vi "ExFileReadNGraphGbl.vi"() -> ()   [LabVIEW 2010]
panel:
  in  "Timeout":i16=1000
  out "FirstRunFlag":bool=TRUE
  in  "Quick Select":u32(knob) min=1 max=1000 scale=0.9..1.0
  in  "Set Position":bool
  out "Update Flag":bool=TRUE
  out "Waveform Graph":u16[](graph)
  in  "Spectrum Number":u32=1 min=1 step=1
  in  "Ending":bool
  in  "Beginning":bool
  out "Frame Number":i32=1
  in  "Backward":bool
  in  "Forward":bool
  in  "Full File Name":path=path "C:/Users/Public/Documents/SIToolKit/LabVIEW/Data Files/HID-LAMP.SPE"
  in  "Stop":bool
  in  "FileType":u32=67371008
  out "error out":errorcluster
  in  "error in (no error)":errorcluster
  # "NOTICE\n\nTHIS VI REQUIRES THAT THE TOOLKIT\nBE UNLOADED BY RUNNING THE\n VI EXCLOSEGLOBALCAM.VI\n BEFORE LEAVING LABVIEW."
  # "ExReadFileNGraphGbl.vi\nThis example will read in a file of the\nselected data type and display all frames.\nWhen finished viewing data, make sure to\nuse the STOP button to close the display."
  # "File Types:\nSPE = 67371008\nTIF   = 67174400\nPMI  = 67436544"
  # "Browse match pattern is set to *.tif.  Modify this if different file type is needed."
  # "This will properly \ndeallocate memory."
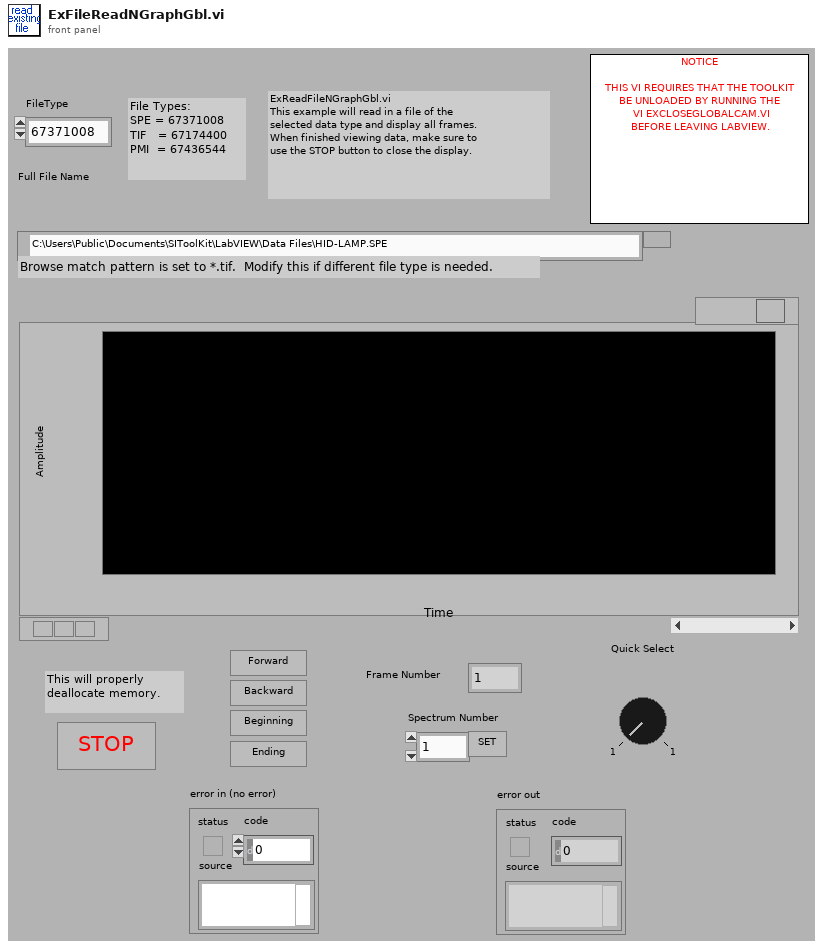
[diagram p1: front panel]
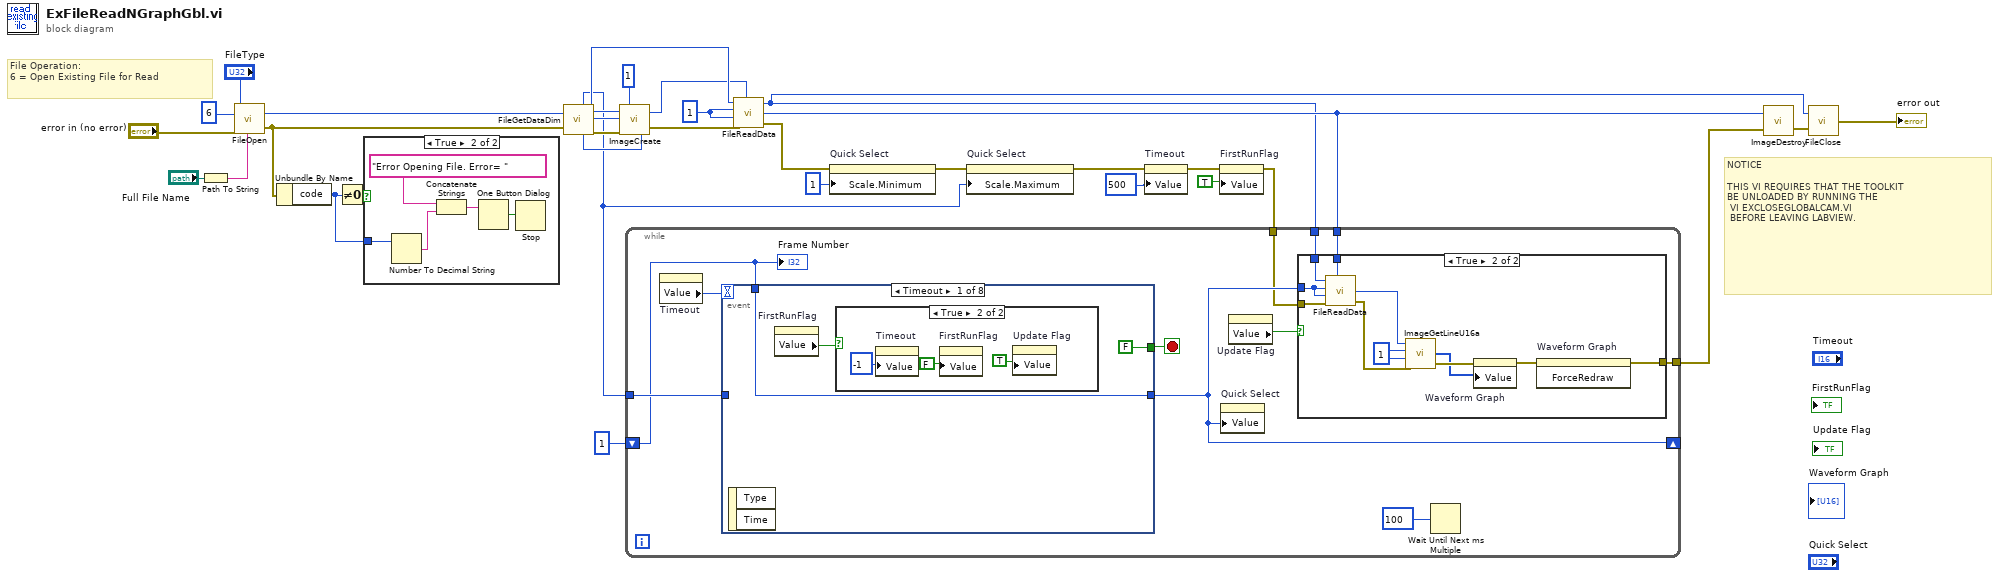
[diagram p0: block diagram]
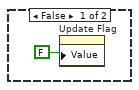
[diagram p3: hidden frame]
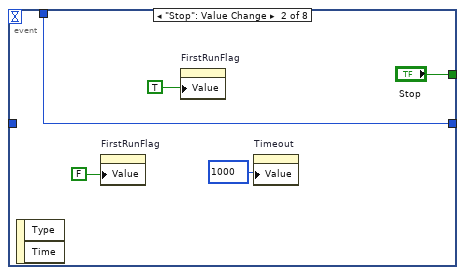
[diagram p4: hidden frame]
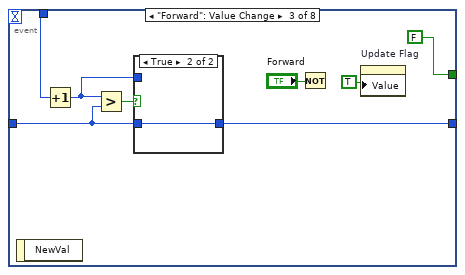
[diagram p5: hidden frame]
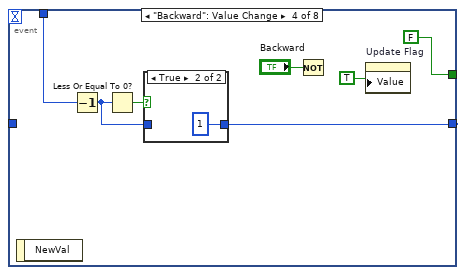
[diagram p7: hidden frame]
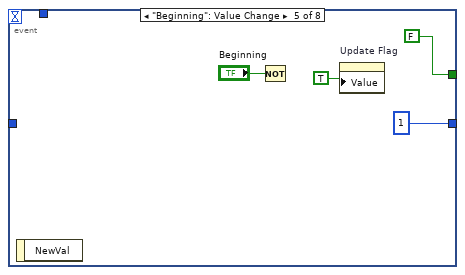
[diagram p9: hidden frame]
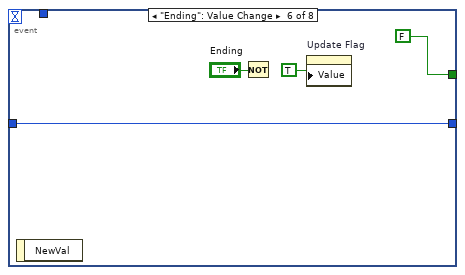
[diagram p10: hidden frame]
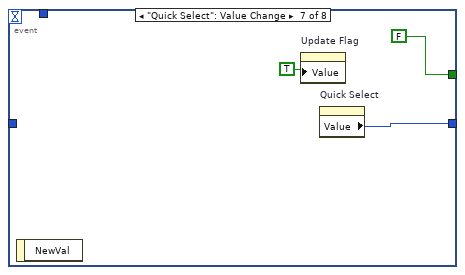
[diagram p11: hidden frame]
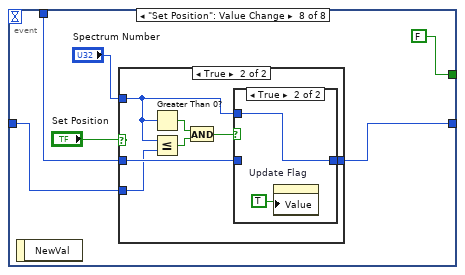
[diagram p12: hidden frame]
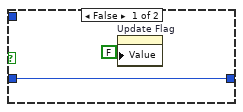
[diagram p13: hidden frame]
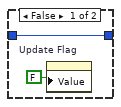
[diagram p14: hidden frame]
diagram:
  w20 = 1
  # "NOTICE\n\nTHIS VI REQUIRES THAT THE TOOLKIT\nBE UNLOADED BY RUNNING THE\n VI EXCLOSEGLOBALCAM.VI\n BEFORE LEAVING LABVIEW."
  # "File Operation:\n6 = Open Existing File for Read"
  n1 = Path To String(path="Full File Name") -> (string=w23:string)
  n2 = call <userlib>:"FileOpen.vi"("error in"="error in (no error)", "File Operations"=u32 6 ("File Operation"), "FileName"=w23, "File Type"="FileType") -> ("error out"=w12:errorcluster, "File Handle"=w17:u32)
  n3 = Unbundle By Name(w12) -> ("code"=w10:i32)
  n4 = Not Equal To 0?(x=w10) -> (x != 0?=w11:bool)
  n5 = case shown="True" w11 {
    tunnel: w10 -> [_ w34]
    frame False {
    }
    frame True {
      n6 = Number To Decimal String(number=w34) -> (decimal integer string=w35:string)  [unwired: 1 in]
      n7 = Concatenate Strings("Error Opening File. Error= ", w35) -> (w37:string)
      n8 = One Button Dialog(message=w37) -> (true=w36:bool)  [unwired: 1 in]
      n9 = Stop(stop? (T)=w36) -> ()
    }
  }
  n10 = call <userlib>:"FileGetDataDim.vi"("File Handle"=w17, "error in"=w12) -> ("Number of Frames"=w6:u32, "Data Type"=w27:u32, "File Handle"=w19:u32, "X dim"=w29:u32, "Y dim"=w28:u32, "error out"=w30:errorcluster)
  n11 = call <userlib>:"ImageCreate.vi"("X dimension"=w29, "Y dimension"=w28, "Data Type"=w27, "error in"=w30, "Number Of Frames"=1) -> ("Image Handle"=w18:u32, "error out"=w13:errorcluster)
  n12 = call <userlib>:"FileReadData.vi"("File Handle"=w19, "Start Frame"=w20, "End Frame"=w20, "error in"=w13, "Image Handle"=w18) -> ("File Handle"=w15:u32, "Image Handle"=w16:u32, "error out"=w8:errorcluster)
  n13 = property on="Quick Select" class="Knob (strict)"(error in=w8, "Scale.Minimum"=1) -> (error out=w9:errorcluster)  [unwired: 1 in, 1 out]
  n14 = property on="Quick Select" class="Knob (strict)"(error in=w9, "Scale.Maximum"=w6) -> (error out=w5:errorcluster)  [unwired: 1 in, 1 out]
  n15 = property on="Timeout" class="DigNum (strict)"(error in=w5, "Value"=500) -> (error out=w3:errorcluster)  [unwired: 1 in, 1 out]
  n16 = property on="FirstRunFlag" class="Bool (strict)"(error in=w3, "Value"=TRUE) -> (error out=w2:errorcluster)  [unwired: 1 in, 1 out]
  n17 = while {
    shift-right: [w42] -> _
    shift-left: 1 -> [w44]
    tunnel: w2 -> [w39]
    tunnel: w15 -> [w48]
    tunnel: w16 -> [w47]
    tunnel: [w49] -> w14
    tunnel: w6 -> [w45]
    stop <- w43 stop-if-true
    n18 = property on="Timeout" class="DigNum (strict)"() -> ("Value"=w41:i16)  [unwired: 2 in, 2 out]
    n19 = event shown="[0] Timeout" {
      selector: _ -> [_ _ _ _ _ _ _ _]
      dyn-events: _ -> [_ _ _ _ _ _ _ _]
      timeout: w41 -> [_ _ _ _ _ _ _ _]
      tunnel: w45 -> [_ _ w67 _ _ w87 _ w96]
      tunnel: w44 -> [w52 w60 w66 w76 _ _ _ w95]
      tunnel: [w52 w60 w65 w75 1 w87 w90 w93] -> w42
      tunnel: [FALSE "Stop" FALSE FALSE FALSE FALSE FALSE FALSE] -> w43
      event Timeout {
        n20 = event-data() -> ()  [unwired: 1 in, 2 out]
        n21 = property on="FirstRunFlag" class="Bool (strict)"() -> ("Value"=w50:bool)  [unwired: 2 in, 2 out]
        n22 = case shown="True" w50 {
          frame False {
            n23 = property on="Update Flag" class="Bool (strict)"("Value"=FALSE) -> ()  [unwired: 2 in, 2 out]
          }
          frame True {
            n24 = property on="Timeout" class="DigNum (strict)"("Value"=-1) -> ()  [unwired: 2 in, 2 out]
            n25 = property on="FirstRunFlag" class="Bool (strict)"("Value"=FALSE) -> ()  [unwired: 2 in, 2 out]
            n26 = property on="Update Flag" class="Bool (strict)"("Value"=TRUE) -> ()  [unwired: 2 in, 2 out]
          }
        }
      }
      event "Stop": Value Change {
        n27 = event-data() -> ()  [unwired: 1 in, 2 out]
        n28 = property on="FirstRunFlag" class="Bool (strict)"("Value"=FALSE) -> ()  [unwired: 2 in, 2 out]
        n29 = property on="FirstRunFlag" class="Bool (strict)"("Value"=TRUE) -> ()  [unwired: 2 in, 2 out]
        n30 = property on="Timeout" class="DigNum (strict)"("Value"=1000) -> ()  [unwired: 2 in, 2 out]
      }
      event "Forward": Value Change {
        n31 = event-data() -> ()  [unwired: 1 in, 1 out]
        n32 = Increment(x=w66) -> (x+1=w68:u32)
        n33 = Greater?(x=w68, y=w67) -> (0:w69:bool)
        n34 = case shown="True" w69 {
          tunnel: w67 -> [_ w71]
          tunnel: [w70 w71] -> w65
          tunnel: w68 -> [w70 _]
          frame False {
          }
          frame True {
          }
        }
        n35 = Not(x="Forward") -> ()  [unwired: 1 out]
        n36 = property on="Update Flag" class="Bool (strict)"("Value"=TRUE) -> ()  [unwired: 2 in, 2 out]
      }
      event "Backward": Value Change {
        n37 = event-data() -> ()  [unwired: 1 in, 1 out]
        n38 = Decrement(x=w76) -> (x-1=w77:u32)
        n39 = Less Or Equal To 0?(x=w77) -> (x <= 0?=w78:bool)
        n40 = case shown="True" w78 {
          tunnel: [w79 1] -> w75
          tunnel: w77 -> [w79 _]
          frame False {
          }
          frame True {
          }
        }
        n41 = Not(x="Backward") -> ()  [unwired: 1 out]
        n42 = property on="Update Flag" class="Bool (strict)"("Value"=TRUE) -> ()  [unwired: 2 in, 2 out]
      }
      event "Beginning": Value Change {
        n43 = event-data() -> ()  [unwired: 1 in, 1 out]
        n44 = Not(x="Beginning") -> ()  [unwired: 1 out]
        n45 = property on="Update Flag" class="Bool (strict)"("Value"=TRUE) -> ()  [unwired: 2 in, 2 out]
      }
      event "Ending": Value Change {
        n46 = event-data() -> ()  [unwired: 1 in, 1 out]
        n47 = Not(x="Ending") -> ()  [unwired: 1 out]
        n48 = property on="Update Flag" class="Bool (strict)"("Value"=TRUE) -> ()  [unwired: 2 in, 2 out]
      }
      event "Quick Select": Value Change {
        n49 = event-data() -> ()  [unwired: 1 in, 1 out]
        n50 = property on="Update Flag" class="Bool (strict)"("Value"=TRUE) -> ()  [unwired: 2 in, 2 out]
        n51 = property on="Quick Select" class="Knob (strict)"() -> ("Value"=w90:u32)  [unwired: 2 in, 2 out]
      }
      event "Set Position": Value Change {
        n52 = event-data() -> ()  [unwired: 1 in, 1 out]
        n53 = case shown="True" "Set Position" {
          tunnel: w95 -> [w99 w101]
          tunnel: [w99 w102] -> w93
          tunnel: "Spectrum Number" -> [_ w103]
          tunnel: w96 -> [_ w100]
          frame False {
            n54 = property on="Update Flag" class="Bool (strict)"("Value"=FALSE) -> ()  [unwired: 2 in, 2 out]
          }
          frame True {
            n55 = Greater Than 0?(x=w103) -> (x > 0?=w105:bool)
            n56 = Less Or Equal?(x=w103, y=w100) -> (x <= y?=w104:bool)
            n57 = And(x=w105, y=w104) -> (x .and. y?=w106:bool)
            n58 = case shown="True" w106 {
              tunnel: w103 -> [_ w110]
              tunnel: [w108 w110] -> w102
              tunnel: w101 -> [w108 _]
              frame False {
                n59 = property on="Update Flag" class="Bool (strict)"("Value"=FALSE) -> ()  [unwired: 2 in, 2 out]
              }
              frame True {
                n60 = property on="Update Flag" class="Bool (strict)"("Value"=TRUE) -> ()  [unwired: 2 in, 2 out]
              }
            }
          }
        }
      }
    }
    n61 = property on="Quick Select" class="Knob (strict)"("Value"=w42) -> ()  [unwired: 2 in, 2 out]
    n62 = property on="Update Flag" class="Bool (strict)"() -> ("Value"=w46:bool)  [unwired: 2 in, 2 out]
    n63 = case shown="True" w46 {
      tunnel: [w111 w112] -> w49
      tunnel: w48 -> [_ w120]
      tunnel: w47 -> [_ w119]
      tunnel: w42 -> [_ w114]
      tunnel: w39 -> [w111 w118]
      frame False {
      }
      frame True {
        w116 = 1
        n64 = call <userlib>:"FileReadData.vi"("File Handle"=w120, "Start Frame"=w114, "End Frame"=w114, "error in"=w118, "Image Handle"=w119) -> ("Image Handle"=w121:u32, "error out"=w117:errorcluster)  [unwired: 1 out]
        n65 = call <userlib>:"ImageGetLineU16a.vi"("Data Handle"=w121, "Y Position"=w116, "Z Position"=w116, "error in"=w117) -> ("Array u16"=w115:u16[], "error out"=w122:errorcluster)  [unwired: 1 in, 1 out]
        n66 = property on="Waveform Graph" class="WFGraph (strict)"(error in=w122, "Value"=w115) -> (error out=w113:errorcluster)  [unwired: 1 in, 1 out]
        n67 = invoke on="Waveform Graph" class="WFGraph (strict)" method="ForceRedraw"(error in=w113) -> (error out=w112:errorcluster)  [unwired: 2 in, 2 out]
      }
    }
    n68 = Wait Until Next ms Multiple(millisecond multiple=100) -> ()  [unwired: 1 out]
    "Frame Number" <- w44
  }
  n69 = call <userlib>:"ImageDestroy.vi"("error in"=w14, "Data handle"=w16) -> ("error out"=w25:errorcluster)
  n70 = call <userlib>:"FileClose.vi"("error in"=w25, "File Handle"=w15) -> ("error out"=→"error out":errorcluster)
